vi "Control Switch.vi"(7 "switch queue":refnum<queue>, 8 "error in (no error)":errorcluster, 10 "current time":dbl, 11 "test params":refnum<class "IA Test Parameters.lvclass">) -> (0 "error out":errorcluster)   [LabVIEW 2020]
uses:
  Parameter Class/IA Test Parameters.lvclass
  Hardware/Actuators/Switches/Switch.lvclass
  C:/Users/jharw/Documents/1 Folder to Rule them All/UMD/Inflation-Apparatus/src/Hardware/General Hardware.lvclass
  Parameter Class/IA Test Parameters.lvclass/IA Test Parameters.ctl
  Hardware/Actuators/Switches/Switch.lvclass/Switch.ctl
  Hardware/General Hardware.lvclass/General Hardware.ctl
  Hardware/General Hardware.lvclass
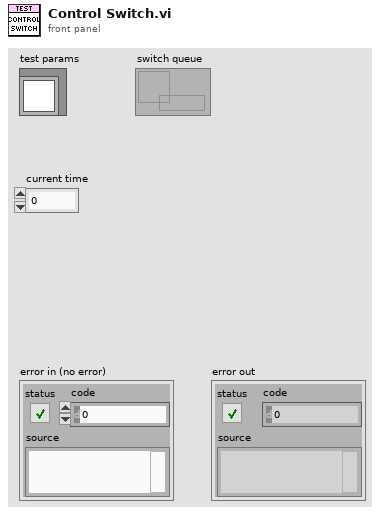
[diagram p1: front panel]
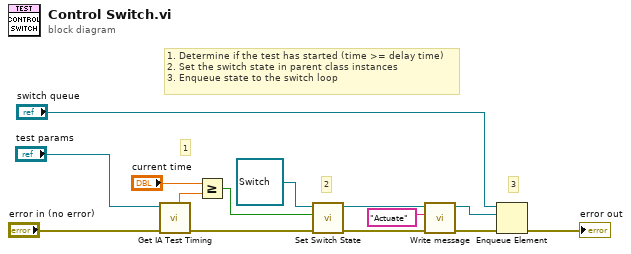
[diagram p0: block diagram]
diagram:
  # "1. Determine if the test has started (time >= delay time)\n2. Set the switch state in parent class instances\n3. Enqueue state to the switch loop"
  # "3"
  # "2"
  # "1"
  n1 = call "Get IA Test Timing.vi"("error in (no error)"="error in (no error)", "IA Test Parameters in"="test params") -> ("error out"=w12:errorcluster, "time delay (sec)"=w9:dbl)  [unwired: 4 in, 4 out]
  n2 = Greater Or Equal?(x="current time", y=w9) -> (x >= y?=w11:bool)
  n3 = call "Set Switch State.vi"("error in (no error)"=w12, "switch state"=w11, "Switch in"=refnum<class "Switch.lvclass"> refnum) -> ("error out"=w4:errorcluster, "Switch out"=w2:refnum<class "Switch.lvclass">)  [unwired: 7 in]
  n4 = call "Write message.vi"("error in (no error)"=w4, "message"="Actuate", "General Hardware in"=w2) -> ("error out"=w3:errorcluster, "General Hardware out"=w1:refnum<class "Switch.lvclass">)  [unwired: 7 in]
  n5 = Enqueue Element(queue="switch queue", element=w1, error in (no error)=w3) -> (error out=→"error out":errorcluster)  [unwired: 1 in, 2 out]
